vi "Read Temperature Set Point (C).vi"(8 "error in (no error)":errorcluster, 11 "Thermal Chamber in":refnum<class "Thermal Chamber.lvclass">) -> (0 "error out":errorcluster, 2 "Temperature Set Point (C)":dbl, 3 "Thermal Chamber out":refnum<class "Thermal Chamber.lvclass">)   [LabVIEW 2026, in "Hardware.lvlib" / "Thermal Chamber.lvclass"]
uses:
  Thermal Chamber.lvclass
  Thermal Chamber.lvclass/Thermal Chamber.ctl
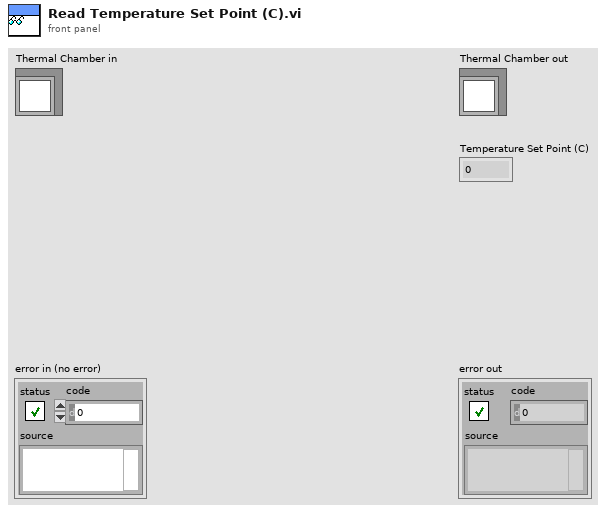
[diagram p1: front panel]
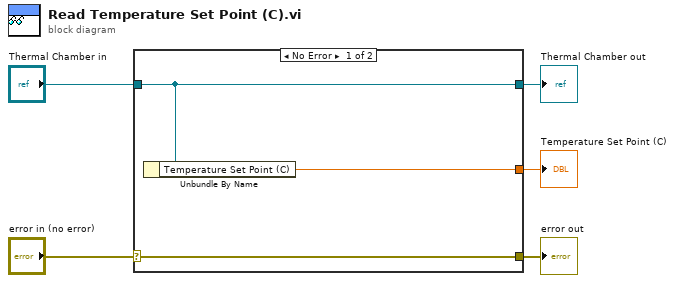
[diagram p0: block diagram]
diagram:
  n1 = case shown="No Error" "error in (no error)" {
    selector: "error in (no error)" -> [w8 w9]
    tunnel: [w8 w9] -> w4
    tunnel: [w7 w10] -> w2
    tunnel: "Thermal Chamber in" -> [w7 w10]
    tunnel: [w6 _] -> w1
    frame No Error {
      n2 = Unbundle By Name(w7) -> ("Temperature Set Point (C)"=w6:dbl)
    }
    frame Error {
    }
  }
  "error out" <- w4
  "Thermal Chamber out" <- w2
  "Temperature Set Point (C)" <- w1
